vi "test-controls.vi"() -> ()   [LabVIEW 2019]
panel:
  in  "Weired/Control/Name=2":dbl
  in  "Weired/Control/Name":dbl
  in  "Time Stamp":timestamp
  in  "Path":path
  out "Signaled":bool
  in  "Cluster":cluster{"Numeric":dbl, "String":string}={"Numeric"=23.0, "String"="aa"}
  in  "StringArray":string[](array[string])=["a", "b", "c"]
  in  "NumericArray":dbl[](array[numeric])=[1.0, 2.0, 3.0]
  in  "Enum":enum16{"zero", "one", "two"}(ring)=enum."two"
  in  "Ring":u16(ring) items=["zero"=0, "two"=2, "four"=4]
  in  "String":string="Hello"
  out "Boolean":bool
  in  "Integer":i64
  in  "Double":dbl
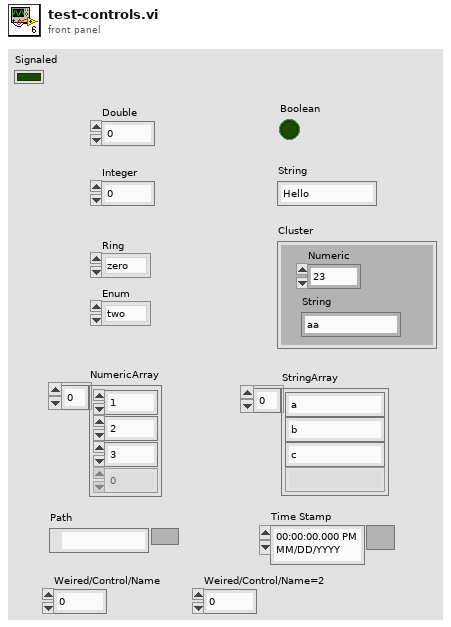
[diagram p1: front panel]
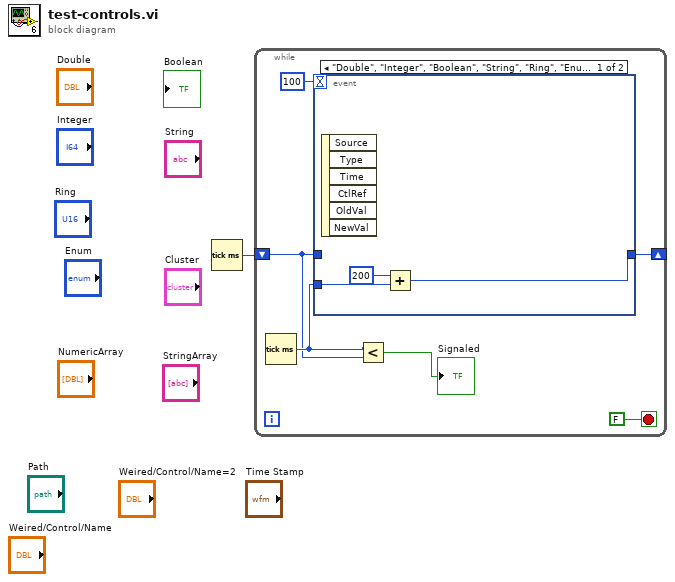
[diagram p0: block diagram]
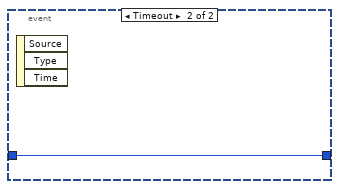
[diagram p2: hidden frame]
diagram:
  n1 = Tick Count (ms)() -> (millisecond timer value=w1:u32)
  n2 = while {
    shift-right: [w6] -> _
    shift-left: w1 -> [w4]
    stop <- FALSE stop-if-true
    n3 = Tick Count (ms)() -> (millisecond timer value=w5:u32)
    n4 = event shown="[0] \"Double\", \"Integer\", \"Boolean\", \"String\", \"Ring\", \"Enum\", \"NumericArray\", \"StringArray\", \"Cluster\", \"Path\", \"Time Stamp\": Value Change" {
      selector: _ -> [_ _]
      dyn-events: _ -> [_ _]
      timeout: 100 -> [_ _]
      tunnel: w5 -> [w10 _]
      tunnel: [w8 w11] -> w6
      tunnel: w4 -> [_ w11]
      event "Double", "Integer", "Boolean", "String", "Ring", "Enum", "NumericArray", "StringArray", "Cluster", "Path", "Time Stamp": Value Change {
        n5 = event-data() -> ()  [unwired: 1 in, 6 out]
        n6 = Add(x=u32 200, y=w10) -> (x+y=w8:u32)
      }
      event Timeout {
        n7 = event-data() -> ()  [unwired: 1 in, 3 out]
      }
    }
    n8 = Less?(x=w5, y=w4) -> (x < y?=→"Signaled":bool)
  }
